vi "ByPntAr2ByLryAr.vi"(11 "Array":cluster{"Image":dbl[][][]}[](array[cluster])) -> (3 "AllStacked":dbl[][][][](array[numeric]))   [LabVIEW 2014]
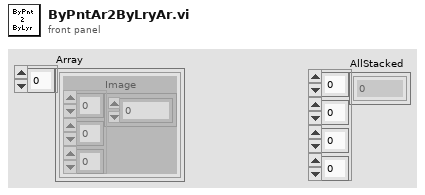
[diagram p1: front panel]
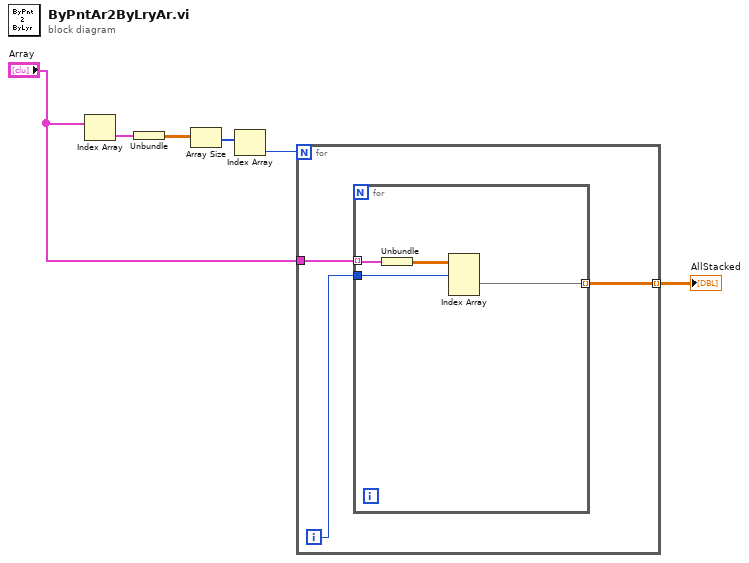
[diagram p0: block diagram]
diagram:
  n1 = Index Array(array="Array") -> (element=w6:cluster{"Image":dbl[][][]})  [unwired: 1 in]
  n2 = Unbundle(w6) -> ("Image"=w5:dbl[][][])
  n3 = Array Size(array=w5) -> (size(s)=w4:i32[])
  n4 = Index Array(array=w4) -> (element=w3:i32)  [unwired: 1 in]
  n5 = for {
    N: w3 -> [_]
    tunnel: "Array" -> [w9]
    tunnel: [w7] -> w1 mode=indexing
    i -> [w8]
    n6 = for {
      tunnel: w9 -> [w13] mode=indexing
      tunnel: w8 -> [w11]
      tunnel: [w10] -> w7 mode=indexing
      n7 = Unbundle(w13) -> ("Image"=w12:dbl[][][])
      n8 = Index Array(array=w12, index (dim 0)=w11) -> (element=w10:dbl[][])  [unwired: 2 in]
    }
  }
  "AllStacked" <- w1
